vi "Test PLC OPC using Datasocket.vi"() -> ()   [LabVIEW 2013]
panel:
  in  "PC_ACK_Read_Tags":dbl
  in  "Invalid_SNo":dbl
  in  "Station_No_Start_Stop_Test":dbl
  in  "Invalid S No":dbl
  in  "Rerun":dbl
  in  "Station_Number":dbl
  in  "Test_Result":dbl
  in  "Serial_Flange_Size":string
  in  "Serial_Displacement_Size":dbl
  in  "Serial_Adapter_Size":dbl
  in  "New_Serial":dbl
  in  "Scan_Trigger":dbl
  in  "Stop_Test":dbl
  in  "Start_Test":dbl
  in  "Task_Available_for_Robot":dbl
  in  "Robot_Available":dbl
  in  "Stop":bool
  # "Run datasocket server in order to run this VI"
  # "Write Tags\nPC Writes to PLC\nPLC can only read these tags"
  # "Read Tags\nPC Reads from PLC"
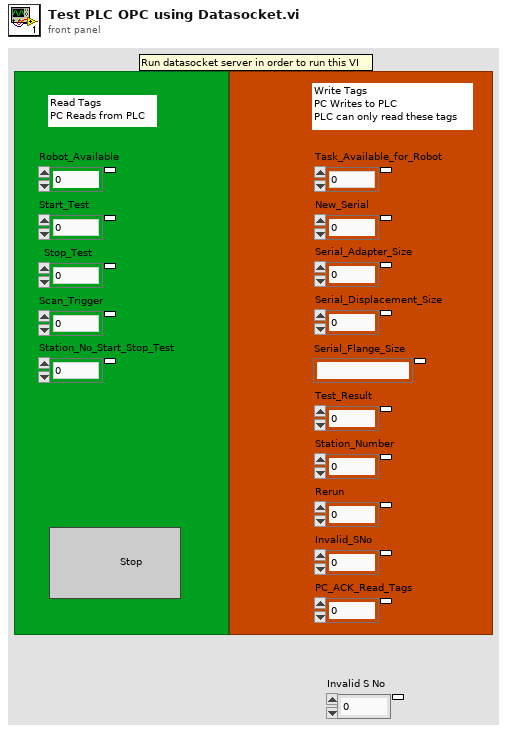
[diagram p1: front panel]
types:
  T1 = enum32{"No PSP", "Read", "Write", "Write & Read"}
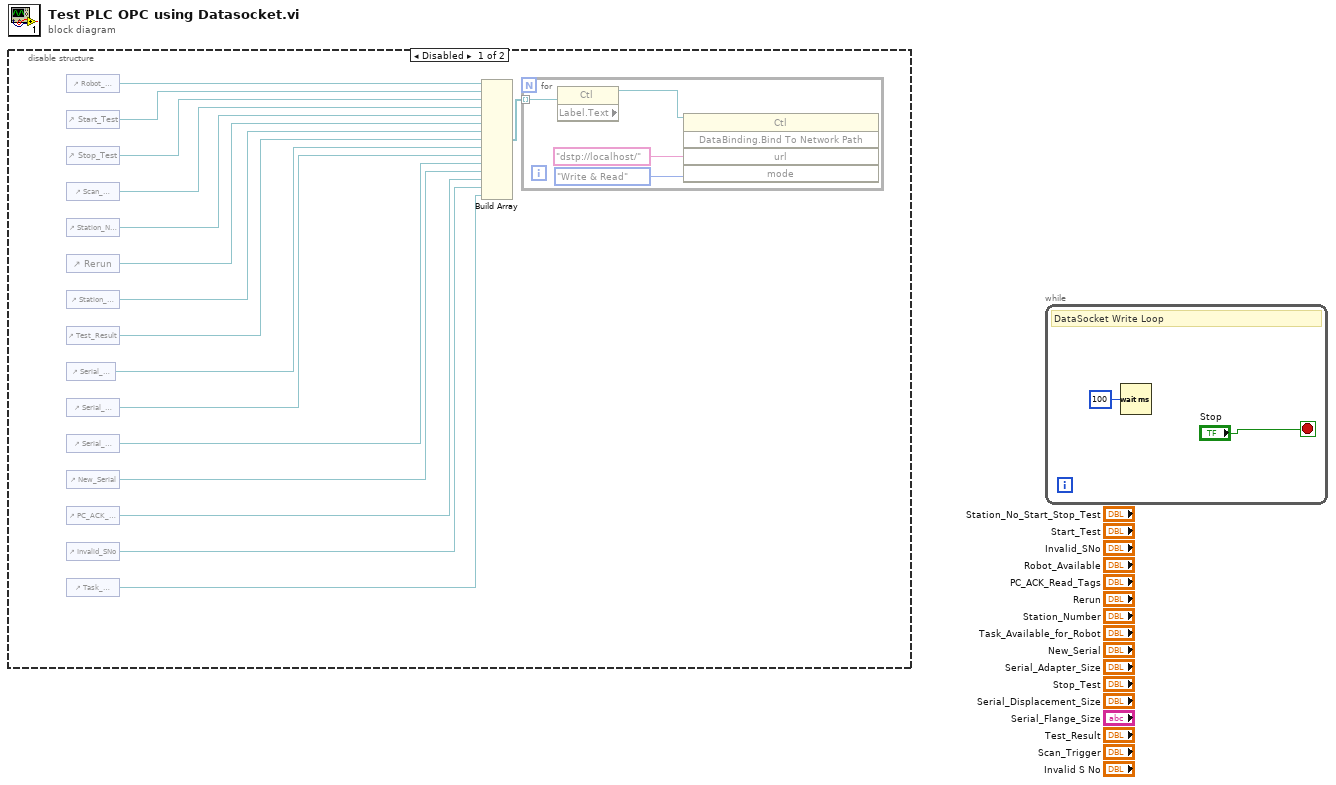
[diagram p0: block diagram]
diagram:
  n1 = disable-structure shown="Disabled" {
    frame Disabled {
      n2 = control-ref of="Robot_Available"() -> (w15:refnum<vi>)
      n3 = control-ref of="Start_Test"() -> (w14:refnum<vi>)
      n4 = control-ref of="Stop_Test"() -> (w13:refnum<vi>)
      n5 = control-ref of="Scan_Trigger"() -> (w12:refnum<vi>)
      n6 = control-ref of="Station_No_Start_Stop_Test"() -> (w11:refnum<vi>)
      n7 = control-ref of="Rerun"() -> (w10:refnum<vi>)
      n8 = control-ref of="Station_Number"() -> (w9:refnum<vi>)
      n9 = control-ref of="Test_Result"() -> (w8:refnum<vi>)
      n10 = control-ref of="Serial_Flange_Size"() -> (w7:refnum<vi>)
      n11 = control-ref of="Serial_Displacement_Size"() -> (w6:refnum<vi>)
      n12 = control-ref of="Serial_Adapter_Size"() -> (w5:refnum<vi>)
      n13 = control-ref of="New_Serial"() -> (w4:refnum<vi>)
      n14 = control-ref of="PC_ACK_Read_Tags"() -> (w3:refnum<vi>)
      n15 = control-ref of="Invalid_SNo"() -> (w2:refnum<vi>)
      n16 = control-ref of="Task_Available_for_Robot"() -> (w1:refnum<vi>)
      n17 = Build Array(w15, w14, w13, w12, w11, w10, w9, w8, w7, w6, w5, w4, w3, w2, w1) -> (w16:refnum<vi>[])
      n18 = for {
        tunnel: w16 -> [w20] mode=indexing
        n19 = property class="Ctl" props=["Label", "Text"](reference=w20) -> (reference out=w17:refnum<vi>)  [unwired: 1 in, 2 out]
        n20 = invoke on="Invoke Node" class="Ctl" method="DataBinding.Bind To Network Path"(reference=w17, "url"="dstp://localhost/" ("URL"), "mode"=T1."Write & Read" ("Mode")) -> ()  [unwired: 2 in, 5 out]
      }
    }
    frame Enabled {
    }
  }
  n21 = while {
    stop <- "Stop" stop-if-true
    # "DataSocket Write Loop"
    n22 = Wait (ms)(milliseconds to wait=u32 100) -> ()  [unwired: 1 out]
  }
